vi "Time 2.1-2.2 compariosn.vi"() -> ()   [LabVIEW 2013]
panel:
  out "Fib":i32
  out "Time3":dbl
  out "Time2":dbl
  out "f(n)":i32
  out "fib(n)":i32
  out "Time1":dbl
  in  "n":i16
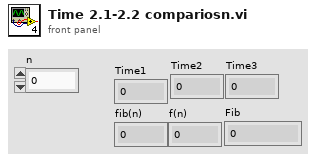
[diagram p1: front panel]
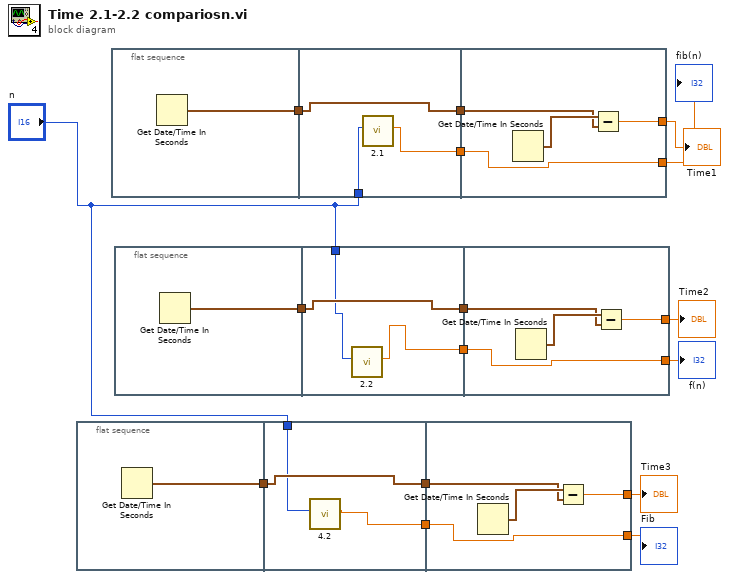
[diagram p0: block diagram]
diagram:
  n1 = flat-sequence {
    tunnel: [w17] -> w10
    tunnel: w10 -> [w20]
    tunnel: [w20] -> w9
    tunnel: [w18] -> w8
    tunnel: "n" -> [w19]
    tunnel: w9 -> [w21]
    tunnel: [w24] -> w3
    tunnel: w8 -> [w23]
    tunnel: [w23] -> w2
    frame #0 {
      n2 = Get Date/Time In Seconds() -> (seconds since 1Jan1904=w17:timestamp)
    }
    frame #1 {
      n3 = call "4.2.vi"("Numeric"=w19) -> ("Numeric 2"=w18:dbl)  [unwired: 10 in]
    }
    frame #2 {
      n4 = Get Date/Time In Seconds() -> (seconds since 1Jan1904=w22:timestamp)
      n5 = Subtract(x=w22, y=w21) -> (x-y=w24:dbl)
    }
  }
  n6 = flat-sequence {
    tunnel: [w25] -> w16
    tunnel: "n" -> [w27]
    tunnel: w16 -> [w28]
    tunnel: [w28] -> w15
    tunnel: [w26] -> w14
    tunnel: w15 -> [w29]
    tunnel: [w32] -> w7
    tunnel: w14 -> [w31]
    tunnel: [w31] -> w6
    frame #0 {
      n7 = Get Date/Time In Seconds() -> (seconds since 1Jan1904=w25:timestamp)
    }
    frame #1 {
      n8 = call "2.1.vi"("Numeric"=w27) -> ("Numeric 2"=w26:dbl)  [unwired: 10 in]
    }
    frame #2 {
      n9 = Get Date/Time In Seconds() -> (seconds since 1Jan1904=w30:timestamp)
      n10 = Subtract(x=w30, y=w29) -> (x-y=w32:dbl)
    }
  }
  n11 = flat-sequence {
    tunnel: [w33] -> w13
    tunnel: w13 -> [w36]
    tunnel: [w36] -> w12
    tunnel: [w34] -> w11
    tunnel: "n" -> [w35]
    tunnel: w12 -> [w37]
    tunnel: [w40] -> w4
    tunnel: w11 -> [w39]
    tunnel: [w39] -> w5
    frame #0 {
      n12 = Get Date/Time In Seconds() -> (seconds since 1Jan1904=w33:timestamp)
    }
    frame #1 {
      n13 = call "2.2.vi"("Numeric"=w35) -> ("Numeric 2"=w34:dbl)  [unwired: 10 in]
    }
    frame #2 {
      n14 = Get Date/Time In Seconds() -> (seconds since 1Jan1904=w38:timestamp)
      n15 = Subtract(x=w38, y=w37) -> (x-y=w40:dbl)
    }
  }
  "Time1" <- w7
  "fib(n)" <- w6
  "f(n)" <- w5
  "Time2" <- w4
  "Time3" <- w3
  "Fib" <- w2
